vi "Main_Transmitter_Localtest.vi"(6 "Input Message":i8[](array[numeric]), 7 "Meas Queue Name":string, 8 "error in (no error)":errorcluster, 9 "Waveform Queue Name":string, 10 "Packet Parameters in":T3={"Length of sync sequence (50)"=50, "Number of message bits"=512, "Number of guardbits"=20, "Sync PN sequence order (31)"=31, "Number of header bits"=16, "Packet Pad [samples]"=200}, 11 "QPSK System Parameters":T4={"Samples per Symbol"=8, "symbol map"=[], "Differential PSK"=enum."disable", "PSK type"=0, "M-PSK"=4} {"PSK type" items=["normal", "shifted", "offset"]; "symbol map" format="%.3f"}) -> (0 "error out":errorcluster, 2 "Frame length [samples]":i32)   [LabVIEW 2014]
uses:
  <vilib>/addons/Modulation/Digital/General/MT Generate Bits (Galois, PN Order).vi
  <vilib>/addons/Modulation/Digital/Support/Common/Validators/mod_Generate Bits Validate.vi
  <vilib>/addons/Modulation/Analog/support/mod_Set Error Source.vi
  <vilib>/addons/Modulation/Digital/General/subVIs/mod_Generate Bits PN Sequence.vi
  <instrlib>/niUSRP/niUSRP Write Tx Data (CDB Cluster).vi
  <vilib>/addons/Modulation/Digital/General/MT Format Eye Diagram (complex).vi
  <vilib>/addons/Modulation/niDMT.lvlib
panel:
  in  "output cluster":cluster{i32, i32, dbl, dbl}
  in  "Test Setup":T1={"Packets to send"=100, "Queue Length"=10, "PN sequence order (9)"=9}
  in  "I/Q (I)":enum16{"I", "Q"}(ring) caption="Eye Diagram I/Q"
  out "Eye Diagram":cluster{"t0":dbl, "dt":dbl, "Y":dbl[]}[](graph)
  in  "autoscale":bool
  out "Constellation Graph":T2(graph)
  out "Frame time [ms]":dbl
  out "Packet length [samples]":i32
  out "Effective bit rate [bits/s]":dbl
  out "Real Frames Sent":i32
  out "Blank Frames Sent":i32
  out "Time per packet [ms]":dbl
  in  "stop 2":bool caption="stop"
  in  "Bits per sample":i32=16
  in  "Audio record time/delay (ms)":i32=200
  in  "Audio sample rate (Fs)":i32=6000
  in  "filter parameters":T5={"Alpha"=0.5, "Filter Length"=6, "TX Filter"=enum."Root Raised Cos"} {"Alpha" format="%.2f"}
  in  "USRP IP address":refnum<k15>="192.168.10.1"
  in  "Tx Parameters":T6={"Tx IQ Sampling\nRate [s/sec]"=400000.0, "Tx Frequency [Hz]"=5795000000.0, "Tx Gain [dB]"=0.0, "Tx Antenna"="TX1"} {"Tx Gain [dB]" format="%#.6p"; "Tx Frequency [Hz]" format="%#.6p"; "Tx IQ Sampling\nRate [s/sec]" format="%#.6p"}
  out "Actual Tx Parameters":T6={"Tx IQ Sampling\nRate [s/sec]"=400000.0, "Tx Frequency [Hz]"=915000000.0, "Tx Gain [dB]"=0.0, "Tx Antenna"="TX1"} {"Tx Gain [dB]" format="%#.6p"; "Tx Frequency [Hz]" format="%#.6p"; "Tx IQ Sampling\nRate [s/sec]" format="%#.6p"}
  # "Calculated values"
  # "Measurements"
  # "Graph Setup"
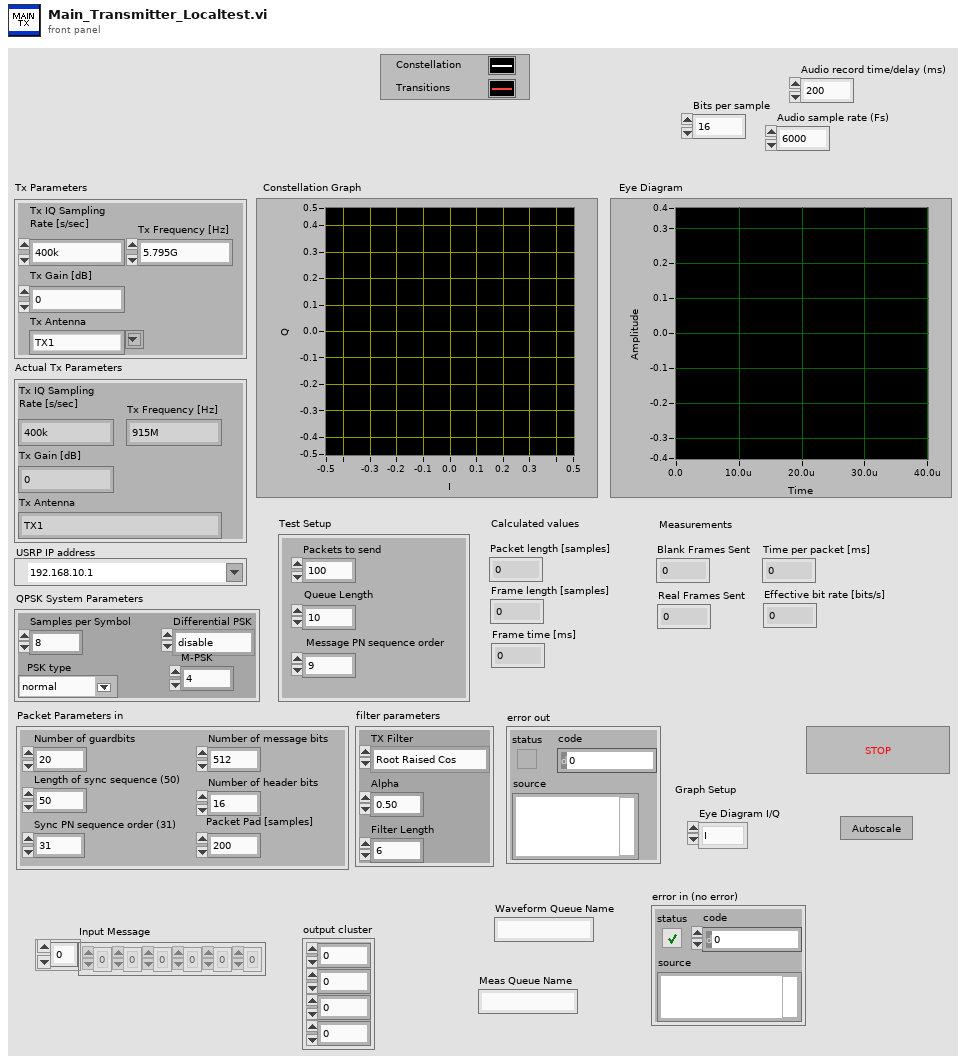
[diagram p1: front panel]
types:
  T1 = cluster{"Packets to send":i32, "Queue Length":i32, "PN sequence order (9)":i32}
  T2 = cluster{"Decimated Array":dbl[], "Decimated Array":dbl[]}[]
  T3 = cluster{"Length of sync sequence (50)":i32, "Number of message bits":i32, "Number of guardbits":i32, "Sync PN sequence order (31)":i32, "Number of header bits":i32, "Packet Pad [samples]":i32}
  T4 = cluster{"Samples per Symbol":i32, "symbol map":cdb[], "Differential PSK":enum16{"disable", "enable"}, "PSK type":u16, "M-PSK":i32}
  T5 = cluster{"Alpha":dbl, "Filter Length":i32, "TX Filter":enum16{"none", "Raised Cosine", "Root Raised Cos", "Gaussian"}}
  T6 = cluster{"Tx IQ Sampling\nRate [s/sec]":dbl, "Tx Frequency [Hz]":dbl, "Tx Gain [dB]":dbl, "Tx Antenna":string}
  T7 = cluster{"samples per symbol (16)":i32, "symbol map":cdb[], "differential PSK":enum16{"disable", "enable"}, "PSK type":u16}
  T8 = cluster{"s? t:f":cluster{"t0":dbl, "dt":dbl, "Y":cdb[]}, i32}
  T9 = typedef "niAMT.lvlib/Complex Data Waveform.ctl" = cluster{"t0":dbl, "dt":dbl, "Y":cdb[]}
  T10 = cluster{"constellation":dbl[], "oversampled data":dbl[]}[]
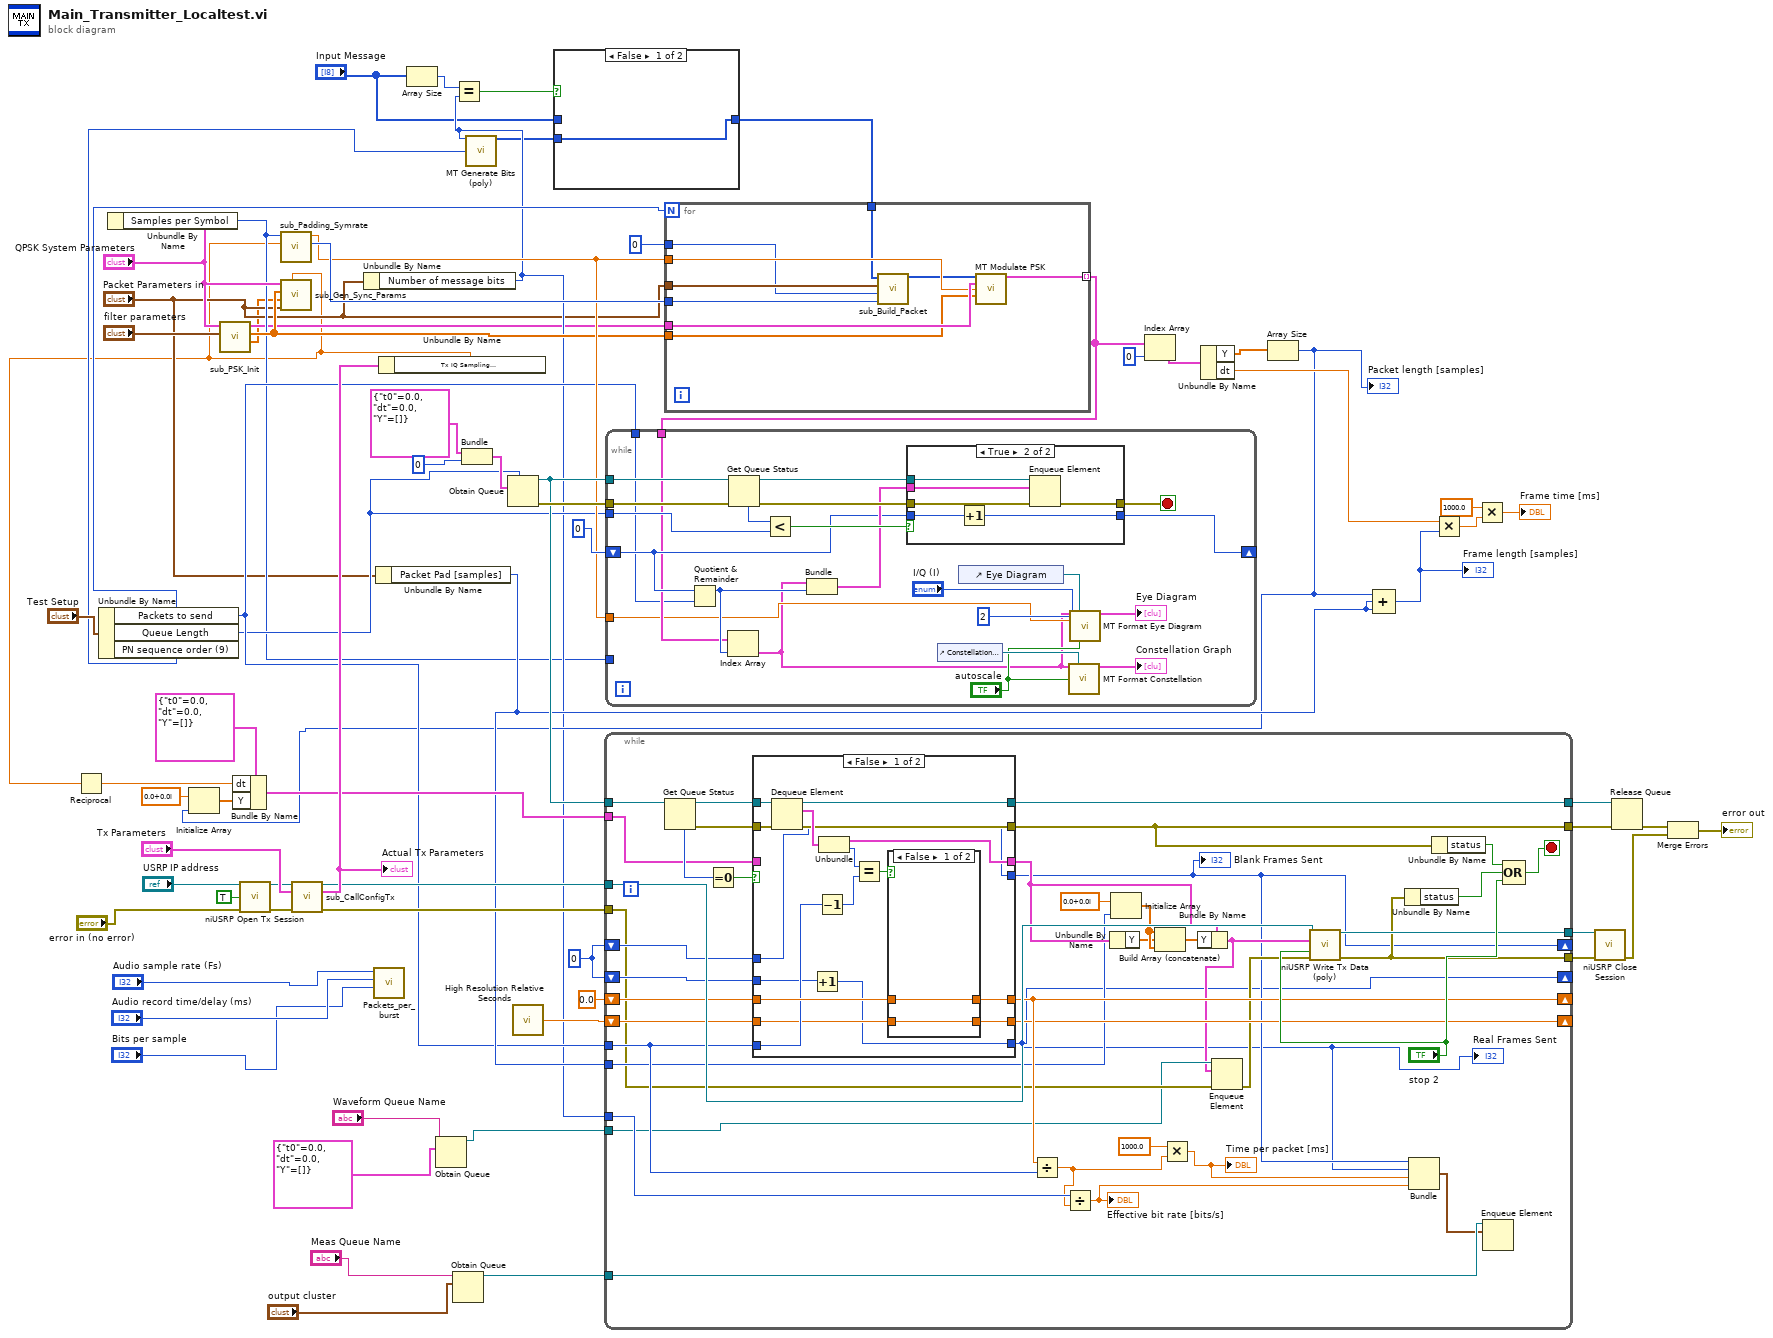
[diagram p0: block diagram]
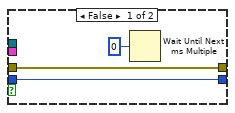
[diagram p3: hidden frame]
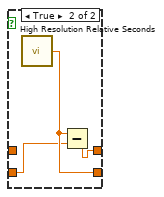
[diagram p4: hidden frame]
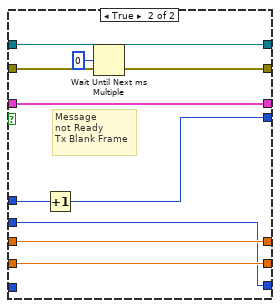
[diagram p5: hidden frame]
diagram:
  w36 = 0
  n1 = Unbundle By Name("Test Setup") -> ("Packets to send"=w23:i32, "Queue Length"=w22:i32, "PN sequence order (9)"=w21:i32)
  n2 = Unbundle By Name("QPSK System Parameters") -> ("Samples per Symbol"=w5:i32)
  n3 = call "sub_PSK_Init.vi"("filter parameters in"="filter parameters", "QPSK System Parameters in"="QPSK System Parameters") -> ("matched filter coefficients"=w2:dbl[], "pulse shaping filter coefficients"=w25:dbl[], "PSK system parameters"=w4:T7)  [unwired: 7 in]
  n4 = call <instrlib>:"niUSRP Open Tx Session.vi"("device names"="USRP IP address", "reset"=TRUE, "error in (no error)"="error in (no error)") -> ("session handle out"=w70:refnum<k15>, "error out"=w69:errorcluster)  [unwired: 11 in]
  n5 = call "sub_CallConfigTx.vi"("session handle"=w70, "Tx Parameters"="Tx Parameters", "error in"=w69) -> ("session handle out"=w64:refnum<k15>, "Actual Tx Parameters"=w65:T6, "error out"=w66:errorcluster)  [unwired: 10 in]
  "Actual Tx Parameters" <- w65
  n6 = Unbundle By Name("Packet Parameters in") -> ("Number of message bits"=w10:i32)
  n7 = call "Packets_per_burst.vi"("Bits per sample"="Bits per sample", "Audio record time/delay (ms)"="Audio record time/delay (ms)", "Audio sample rate (Fs)"="Audio sample rate (Fs)") -> ()  [unwired: 8 in, 1 out]
  n8 = Unbundle By Name("Packet Parameters in") -> ("Packet Pad [samples]"=w27:i32)
  n9 = Unbundle By Name(w65) -> ("Tx IQ Sampling\nRate [s/sec]"=w1:dbl)
  n10 = Reciprocal(x=w1) -> (1/x=w48:dbl)
  n11 = call "sub_Padding_Symrate.vi"("Tx IQ Sampling\nRate [s/sec]"=w1, "Samples per Symbol"=w5) -> ("Padding Bits"=w57:i32, "Symbol Rate"=w26:dbl)  [unwired: 8 in]
  n12 = call "sub_Gen_Sync_Params.vi"("IQ Sampling\nRate [s/sec]"=w1, "Packet Parameters in"="Packet Parameters in", "matched filter coefficients"=w2, "pulse shaping filter coefficients"=w25, "QPSK System Parameters in"="QPSK System Parameters") -> ()  [unwired: 3 in, 4 out]
  n13 = Array Size(array="Input Message") -> (size(s)=w11:i32)
  n14 = Obtain Queue(name (unnamed)="Waveform Queue Name", element data type=cluster{"t0":dbl, "dt":dbl, "Y":cdb[]} {"t0"=0.0, "dt"=0.0, "Y"=[]} ("s? t:f")) -> (queue out=w20:refnum<queue>)  [unwired: 3 in, 2 out]
  n15 = Obtain Queue(name (unnamed)="Meas Queue Name", element data type="output cluster") -> (queue out=w14:refnum<queue>)  [unwired: 3 in, 2 out]
  n16 = Equal?(x=w11, y=w10) -> (x = y?=w9:bool)
  n17 = Bundle("s? t:f"=cluster{"t0":dbl, "dt":dbl, "Y":cdb[]} {"t0"=0.0, "dt"=0.0, "Y"=[]}, 0) -> (w55:T8)  [unwired: 1 in]
  n18 = call-poly <vilib>:"MT Generate Bits (poly).vi"("total bits (128)"=w10, "PN sequence order (9)"=w21) -> ("output bit stream"=w6:i8[])  [unwired: 11 in, 2 out]
  n19 = Obtain Queue(max queue size (-1, unlimited)=w22, element data type=w55) -> (queue out=w51:refnum<queue>, error out=w53:errorcluster)  [unwired: 3 in, 1 out]
  n20 = call <vilib>:"High Resolution Relative Seconds.vi"() -> ("relative seconds"=w38:dbl)
  n21 = case shown="False" w9 {
    tunnel: [w72 w73] -> w8
    tunnel: "Input Message" -> [_ w73]
    tunnel: w6 -> [w72 _]
    frame False {
    }
    frame True {
    }
  }
  n22 = for {
    N: w23 -> [_]
    tunnel: w57 -> [w82]
    tunnel: w8 -> [w77]
    tunnel: w4 -> [w81]
    tunnel: w26 -> [w80]
    tunnel: w25 -> [w79]
    tunnel: [w75] -> w35 mode=indexing
    tunnel: "Packet Parameters in" -> [w78]
    tunnel: i16 0 -> [w76]
    n23 = call "sub_Build_Packet.vi"("Cyclic Padding Bits"=w82, "Packet number"=w76, "Packet Parameters in"=w78, "Input Message"=w77) -> ("Packet out"=w74:i8[])  [unwired: 7 in]
    n24 = call <vilib>:"MT Modulate PSK.vi"("input bit stream"=w74, "PSK system parameters"=w81, "symbol rate (Hz)"=w80, "pulse shaping filter coefficients"=w79) -> ("output complex waveform"=w75:T9)  [unwired: 9 in, 2 out]
  }
  n25 = while {
    tunnel: w51 -> [w99]
    tunnel: w53 -> [w98]
    tunnel: w22 -> [w97]
    tunnel: w35 -> [w94]
    tunnel: w5 -> [_]
    tunnel: w23 -> [w93]
    shift-right: [w92] -> _
    shift-left: 0 -> [w96]
    tunnel: w26 -> [w85]
    stop <- w95 stop-if-true
    n26 = Quotient & Remainder(x=w96, y=w93) -> (x-y*floor(x/y)=w100:i32)  [unwired: 1 out]
    n27 = Index Array(array=w94, index=w100) -> (element=w83:T9)
    n28 = Get Queue Status(queue=w99, error in (no error)=w98) -> (queue out=w105:refnum<queue>, error out=w102:errorcluster, # elements in queue=w104:i32)  [unwired: 1 in, 5 out]
    n29 = Less?(x=w104, y=w97) -> (x < y?=w103:bool)
    n30 = Bundle("output complex waveform"=w83, w100) -> (w101:cluster{"output complex waveform":T9, i32})  [unwired: 1 in]
    n31 = case shown="True" w103 {
      tunnel: w102 -> [w106 w114]
      tunnel: w105 -> [_ w113]
      tunnel: [w106 w112] -> w95
      tunnel: w101 -> [_ w111]
      tunnel: w96 -> [w108 w110]
      tunnel: [w108 w109] -> w92
      frame False {
        n32 = Wait Until Next ms Multiple(millisecond multiple=u32 0) -> ()  [unwired: 1 out]
      }
      frame True {
        n33 = Increment(x=w110) -> (x+1=w109:i32)
        n34 = Enqueue Element(queue=w113, element=w111, error in (no error)=w114) -> (error out=w112:errorcluster)  [unwired: 1 in, 2 out]
      }
    }
    n35 = control-ref of="Constellation Graph"() -> (w88:refnum<vi>)
    n36 = control-ref of="Eye Diagram"() -> (w90:refnum<vi>)
    n37 = call <vilib>:"MT Format Constellation.vi"("waveform"=w83, "constellation reference"=w88, "autoscale"="autoscale") -> ("constellation graph"=→"Constellation Graph":T10)  [unwired: 2 in, 10 out]
    n38 = call-poly <vilib>:"MT Format Eye Diagram.vi"("waveform"=w83, "eye diagram reference"=w90, "symbol rate (Hz)"=w85, "eye length"=2, "I/Q (I)"="I/Q (I)", "autoscale"="autoscale") -> ("eye diagram"=→"Eye Diagram":cluster{"t0":dbl, "dt":dbl, "Y":dbl[]}[])  [unwired: 1 in, 8 out]
  }
  n39 = Index Array(array=w35, index=0) -> (element=w33:T9)
  n40 = Unbundle By Name(w33) -> ("Y"=w32:cdb[], "dt"=w31:dbl)
  n41 = Array Size(array=w32) -> (size(s)=w12:i32)
  "Packet length [samples]" <- w12
  n42 = Initialize Array(cdb 0.0+0.0i ("element"), w12) -> (w49:cdb[])
  n43 = Bundle By Name(cluster=cluster{"t0":dbl, "dt":dbl, "Y":cdb[]} {"t0"=0.0, "dt"=0.0, "Y"=[]} ("s? t:f"), "dt"=w48, "Y"=w49) -> (w46:cluster{"t0":dbl, "dt":dbl, "Y":cdb[]})
  n44 = while {
    tunnel: w66 -> [w123]
    tunnel: w64 -> [w146]
    tunnel: w51 -> [w148]
    tunnel: w46 -> [w147]
    tunnel: [w144] -> w42
    tunnel: [w143] -> w41
    tunnel: [w142] -> w40
    tunnel: [w141] -> w39
    shift-right: [w139] -> _
    shift-left: 0.0 -> [w140]
    tunnel: w23 -> [w138]
    shift-right: [w137] -> _
    shift-left: w38 -> [w136]
    shift-right: [w120] -> _
    shift-left: w36 -> [w135]
    shift-right: [w119] -> _
    shift-left: w36 -> [w134]
    tunnel: w10 -> [w133]
    tunnel: w27 -> [w127]
    tunnel: w20 -> [w122]
    tunnel: w14 -> [w116]
    stop <- w145 stop-if-true
    n45 = Get Queue Status(queue=w148) -> (queue out=w153:refnum<queue>, error out=w152:errorcluster, # elements in queue=w155:i32)  [unwired: 2 in, 5 out]
    n46 = Equal To 0?(x=w155) -> (x = 0?=w154:bool)
    n47 = case shown="False" w154 {
      tunnel: w147 -> [_ w186]
      tunnel: [w168 w186] -> w128
      tunnel: [w172 w184] -> w144
      tunnel: [w167 w185] -> w143
      tunnel: w153 -> [w171 w184]
      tunnel: w152 -> [w170 w185]
      tunnel: w140 -> [w164 w182]
      tunnel: [w163 w182] -> w139
      tunnel: w138 -> [w161 _]
      tunnel: [w160 w181] -> w137
      tunnel: w136 -> [w159 w181]
      tunnel: w135 -> [w158 w180]
      tunnel: [w158 w179] -> w120
      tunnel: w134 -> [w157 w178]
      tunnel: [w156 w178] -> w119
      frame False {
        n48 = Dequeue Element(queue=w171, error in (no error)=w170) -> (queue out=w172:refnum<queue>, element=w169:T8, error out=w167:errorcluster)  [unwired: 1 in, 1 out]
        n49 = Increment(x=w157) -> (x+1=w156:i32)
        n50 = Decrement(x=w161) -> (x-1=w162:i32)
        n51 = Unbundle(w169) -> ("s? t:f"=w168:cluster{"t0":dbl, "dt":dbl, "Y":cdb[]}, w165:i32)
        n52 = Equal?(x=w165, y=w162) -> (x = y?=w166:bool)
        n53 = case shown="False" w166 {
          tunnel: w164 -> [w173 _]
          tunnel: [w173 w177] -> w163
          tunnel: [w174 w176] -> w160
          tunnel: w159 -> [w174 w175]
          frame False {
          }
          frame True {
            n54 = call <vilib>:"High Resolution Relative Seconds.vi"() -> ("relative seconds"=w176:dbl)
            n55 = Subtract(x=w176, y=w175) -> (x-y=w177:dbl)
          }
        }
      }
      frame True {
        # "Message\nnot Ready\nTx Blank Frame"
        n56 = Increment(x=w180) -> (x+1=w179:i32)
        n57 = Wait Until Next ms Multiple(millisecond multiple=u32 0) -> ()  [unwired: 1 out]
      }
    }
    "Blank Frames Sent" <- w120
    "Real Frames Sent" <- w119
    n58 = Divide(x=w139, y=w138) -> (x/y=w125:dbl)
    n59 = Divide(x=w133, y=w125) -> (x/y=w117:dbl)
    "Effective bit rate [bits/s]" <- w117
    n60 = Unbundle By Name(w128) -> ("Y"=w129:cdb[])
    n61 = Initialize Array(cdb 0.0+0.0i ("element"), w127) -> (w130:cdb[])
    n62 = Build Array (concatenate)(w130, w129, w130) -> (w132:cdb[])
    n63 = Multiply(x=1000.0, y=w125) -> (x*y=w118:dbl)
    "Time per packet [ms]" <- w118
    n64 = Bundle By Name(cluster=w128, "Y"=w132) -> (w121:cluster{"t0":dbl, "dt":dbl, "Y":cdb[]})
    n65 = Enqueue Element(queue=w122, element=w121, error in (no error)=w123) -> (error out=w124:errorcluster)  [unwired: 1 in, 2 out]
    n66 = call-poly <instrlib>:"niUSRP Write Tx Data (poly).vi"("session handle"=w146, "data"=w121, "end of data?"="stop 2", "error in (no error)"=w124) -> ("session handle out"=w142:refnum<k15>, "error out"=w141:errorcluster)  [unwired: 10 in]
    n67 = Unbundle By Name(w141) -> ("status"=w151:bool)
    n68 = Bundle(w120, w119, w118, w117) -> (w115:cluster{i32, i32, dbl, dbl})  [unwired: 1 in]
    n69 = Unbundle By Name(w143) -> ("status"=w149:bool)
    n70 = Enqueue Element(queue=w116, element=w115) -> ()  [unwired: 2 in, 3 out]
    n71 = Compound Arithmetic op=OR(w149, w151, "stop 2") -> (w145:bool)
  }
  n72 = Compound Arithmetic op=ADD(w12, w27, w27) -> (w13:i32)
  "Frame length [samples]" <- w13
  n73 = Multiply(x=w31, y=w13) -> (x*y=w30:dbl)
  n74 = Multiply(x=1000.0, y=w30) -> (x*y=→"Frame time [ms]":dbl)
  n75 = call <instrlib>:"niUSRP Close Session.vi"("session handle"=w40, "error in (no error)"=w39) -> ("error out"=w44:errorcluster)  [unwired: 13 in]
  n76 = Release Queue(queue=w42, error in (no error)=w41) -> (error out=w45:errorcluster)  [unwired: 3 out]
  n77 = Merge Errors(w45, w44) -> (→"error out":errorcluster)
